vi "Moving_Statistic_Initialize.vi"(8 "error in (no error)":errorcluster, 10 "Window":dbl, 11 "Moving_Mean in":refnum<class "Moving_Statistic.lvclass">) -> (0 "error out":errorcluster, 3 "Moving_Mean out":refnum<class "Moving_Statistic.lvclass">)   [LabVIEW 2021, in "Moving_Statistic.lvclass"]
uses:
  Moving_Statistic.lvclass
  Moving_Statistic.lvclass/Moving_Statistic.ctl
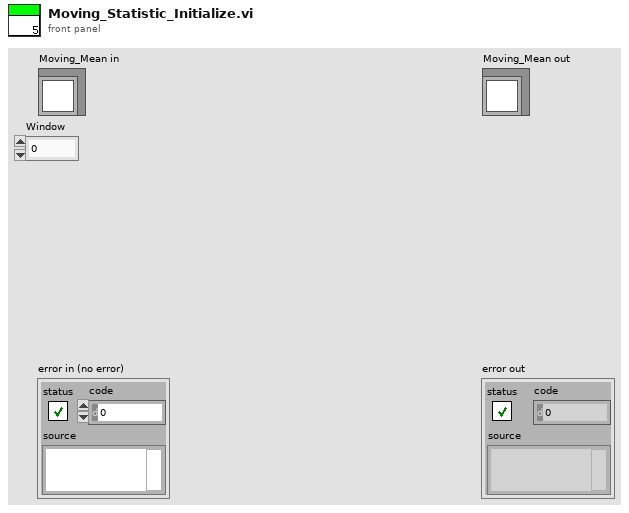
[diagram p1: front panel]
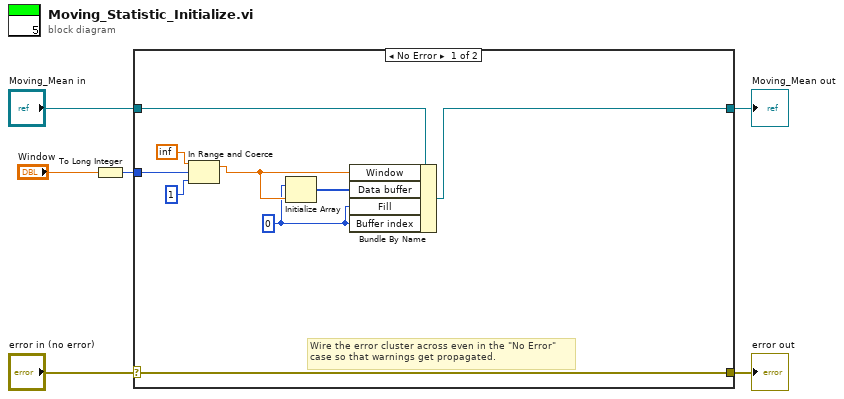
[diagram p0: block diagram]
diagram:
  n1 = To Long Integer(number="Window") -> (32bit integer=w1:i32)
  n2 = case shown="No Error" "error in (no error)" {
    selector: "error in (no error)" -> [w15 w17]
    tunnel: [w15 w17] -> w5
    tunnel: [w13 w16] -> w3
    tunnel: "Moving_Mean in" -> [w14 w16]
    tunnel: w1 -> [w11 _]
    frame No Error {
      w7 = 0 ("Fill")
      # "Wire the error cluster across even in the \"No Error\"\ncase so that warnings get propagated."
      n3 = In Range and Coerce(upper limit=inf, x=w11, lower limit=1) -> (coerced(x)=w10:dbl)  [unwired: 1 out]
      n4 = Initialize Array(w7, w10) -> (w12:i32[])
      n5 = Bundle By Name(cluster=w14, "Window"=w10, "Data buffer"=w12, "Fill"=w7, "Buffer index"=w7) -> (w13:refnum<class "Moving_Statistic.lvclass">)
    }
    frame Error {
    }
  }
  "error out" <- w5
  "Moving_Mean out" <- w3
